vi "Actor Core.vi"(8 "error in":errorcluster, 11 "Timing Engine in":refnum<class "Timing Engine.lvclass">) -> (0 "error out":errorcluster, 3 "Actor out":refnum<class "Actor.lvclass">)   [LabVIEW 2016, in "Assert API Components.lvlib" / "Assert Display.lvlib" / "Timing Engine.lvlib" / "Timing Engine.lvclass"]
doc: "(<B>Filename</B>: Actor Framework.lvlib:Actor.lvclass:Actor Core.vi)\n\nReceives messages to the actor, reacts to them, and initiates any error handling that may shut the actor down.\n\nDescendant classes may override this VI to append parallel tasks for the actor to complete while it handles messages. Overrides use the Call Parent Method node."
uses:
  Timing Engine.lvclass
  C:/Users/ukhornp/Documents/Work/Projects/actor_assert_api/Core/Base UI Actor/Base UI Actor/Base UI Actor.lvclass
  C:/Program Files (x86)/National Instruments/LabVIEW 2016/vi.lib/ActorFramework/Actor/Actor.lvclass
  <vilib>/ActorFramework/Actor/Actor.lvclass
  <vilib>/ActorFramework/Actor/Actor.lvclass/Actor.ctl
  Base UI Actor/Base UI Actor/Base UI Actor.lvclass/Base UI Actor.ctl
  Timing Engine.lvclass/Timing Engine.ctl
  <vilib>/ActorFramework/Message Enqueuer/Message Enqueuer.lvclass/Message Enqueuer.ctl
  <vilib>/ActorFramework/Message Enqueuer/Enqueue.vi
  Timing Engine Messages/Update Msg/Update Msg.lvclass
  C:/Program Files (x86)/National Instruments/LabVIEW 2016/vi.lib/ActorFramework/Message/Message.lvclass
  <vilib>/Utility/LVClass/Get LV Class Name.vi
  <resource>/AFDebug/Generate Trace for Message.vi
  <vilib>/ActorFramework/Message Priority Queue/Priority Enqueue.vi
  Base UI Actor/Base UI Actor/Base UI Actor.lvclass
panel:
  out "Count":i32
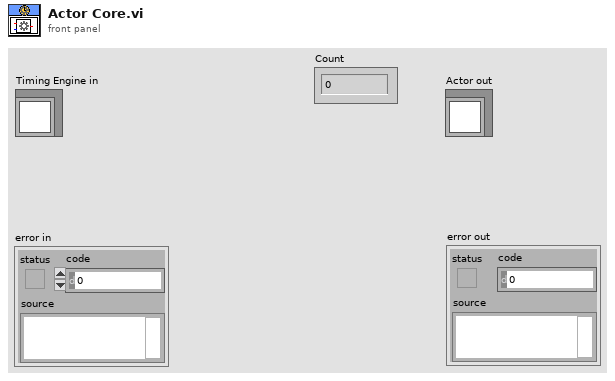
[diagram p1: front panel]
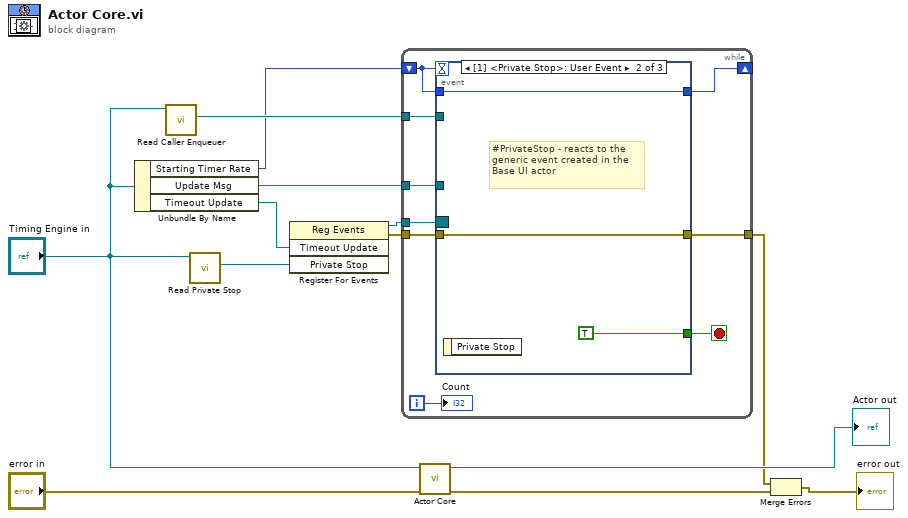
[diagram p0: block diagram]
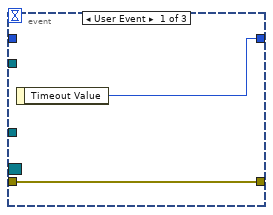
[diagram p2: hidden frame]
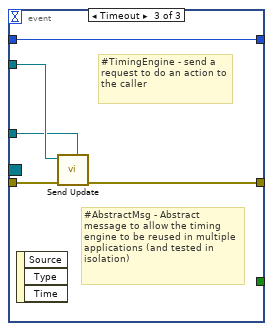
[diagram p3: hidden frame]
diagram:
  n1 = Unbundle By Name("Timing Engine in") -> ("Starting Timer Rate"=w1:i32, "Update Msg"=w2:refnum<class "Update Msg.lvclass">, "Timeout Update"=w11:refnum<user-event>)
  n2 = call <vilib>:"Read Caller Enqueuer.vi"("Actor"="Timing Engine in") -> ("Caller Enqueuer"=w3:refnum<class "Message Enqueuer.lvclass">)  [unwired: 10 in]
  n3 = call "Read Private Stop.vi"("Base UI Actor in"="Timing Engine in") -> ("Private Stop"=w9:refnum<user-event>)  [unwired: 10 in]
  n4 = register-events(w11, w9) -> (reference out=w10:refnum<event-registration>, error out=w8:errorcluster)  [unwired: 2 in]
  n5 = while {
    shift-right: [w21] -> _
    shift-left: w1 -> [w20]
    tunnel: w10 -> [w22]
    tunnel: w8 -> [w18]
    tunnel: [w17] -> w5
    tunnel: w3 -> [w15]
    tunnel: w2 -> [w14]
    i -> [w16]
    stop <- w19 stop-if-true
    n6 = event shown="[1] <Private Stop>: User Event" {
      selector: w22 -> [_ _ _]
      dyn-events: _ -> [_ _ _]
      timeout: w20 -> [_ _ _]
      tunnel: [w24 w25 w32] -> w21
      tunnel: w20 -> [_ w25 w32]
      tunnel: [_ TRUE _] -> w19
      tunnel: w18 -> [w23 w27 w31]
      tunnel: [w23 w27 w30] -> w17
      tunnel: w15 -> [_ _ w29]
      tunnel: w14 -> [_ _ w28]
      event User Event {
        n7 = event-data() -> ("Timeout Value"=w24:i32)  [unwired: 1 in]
      }
      event User Event {
        # "#PrivateStop - reacts to the generic event created in the Base UI actor"
        n8 = event-data() -> ()  [unwired: 1 in, 1 out]
      }
      event Timeout {
        # "#TimingEngine - send a request to do an action to the caller"
        # "#AbstractMsg - Abstract message to allow the timing engine to be reused in multiple applications (and tested in isolation)"
        n9 = event-data() -> ()  [unwired: 1 in, 3 out]
        n10 = call "Send Update.vi"("Message Type"=w28, "error in (no error)"=w31, "Message Enqueuer"=w29) -> ("error out"=w30:errorcluster)  [unwired: 7 in, 1 out]
      }
    }
    "Count" <- w16
  }
  n11 = call-parent "Actor Core.vi"("error in"="error in", "Actor in"="Timing Engine in") -> ("error out"=w13:errorcluster, "Actor out"=→"Actor out":refnum<class "Actor.lvclass">)  [unwired: 8 in]
  n12 = Merge Errors(w5, w13) -> (→"error out":errorcluster)
